vi "Update.vi"(8 "error in (no error)":errorcluster, 10 "user info list":T1, 11 "[V] User List in":refnum<class "[V] User List.lvclass">) -> (0 "error out":errorcluster, 3 "[V] User List out":refnum<class "[V] User List.lvclass">)   [LabVIEW 2020, in "[V] User List.lvlib" / "[V] User List.lvclass"]
uses:
  [V] User List.lvclass
  Control/User Info List.ctl
  [V] User List.lvclass/[V] User List.ctl
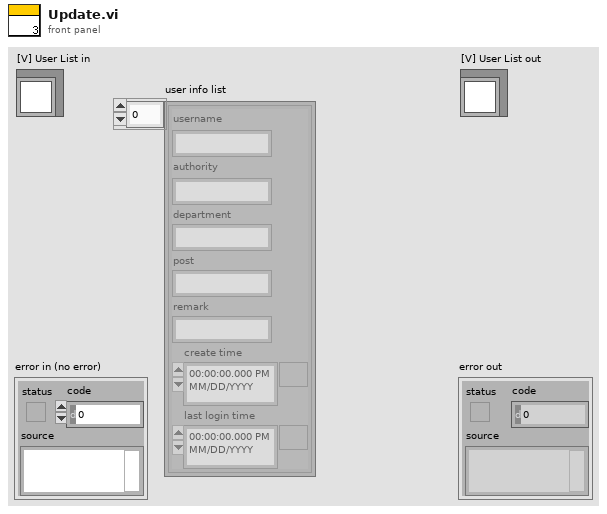
[diagram p1: front panel]
types:
  T1 = typedef "[V] User List.lvlib/[V] User List.lvclass/User Info List.ctl" = cluster{"username":string, "authority":string, "department":string, "post":string, "remark":string, "create time":timestamp, "last login time":timestamp}[]
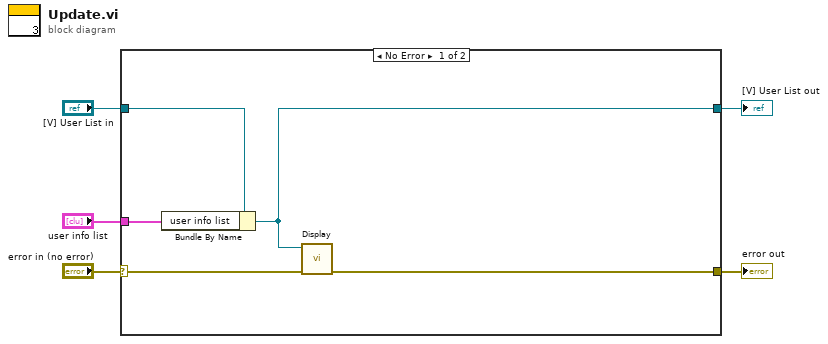
[diagram p0: block diagram]
diagram:
  n1 = case shown="No Error" "error in (no error)" {
    selector: "error in (no error)" -> [w8 w12]
    tunnel: [w6 w12] -> w4
    tunnel: [w7 w11] -> w2
    tunnel: "[V] User List in" -> [w10 w11]
    tunnel: "user info list" -> [w9 _]
    frame No Error {
      n2 = Bundle By Name(cluster=w10, "user info list"=w9) -> (w7:refnum<class "[V] User List.lvclass">)
      n3 = call "Display.vi"("error in (no error)"=w8, "[V] User List in"=w7) -> ("error out"=w6:errorcluster)  [unwired: 8 in, 1 out]
    }
    frame Error {
    }
  }
  "error out" <- w4
  "[V] User List out" <- w2
